vi "Write Pulse Recorder Configuration.vi"(8 "error in (no error)":errorcluster, 10 "Configuration":T1={"Pre-trigger duration"=0.01, "Post-trigger duration"=0.1, "Rate"=1000000.0, "Ranges"=[10.0], "Re-name channels"=[], "Active channels"="0:1", "External clock"=FALSE} {"Rate" format="%#_8pHz"; "Post-trigger duration" format="%#_6ps"; "Pre-trigger duration" format="%#_6ps"; "Ranges" format="%#_6pV"}, 11 "RP I-V in":refnum<class "RP I-V.lvclass">) -> (0 "error out":errorcluster, 3 "RP I-V out":refnum<class "RP I-V.lvclass">)   [LabVIEW 2016, in "RP I-V.lvclass"]
uses:
  RP I-V.lvclass
  NHMFL_Core/Libraries/Instruments/Pulse Driver/Pusle Driver Configuration.ctl
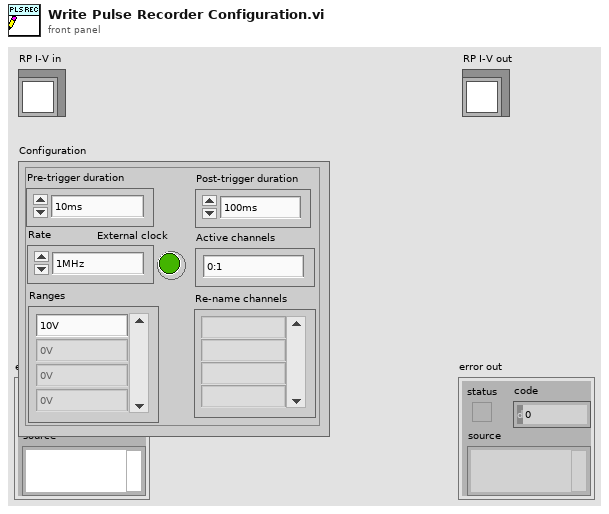
[diagram p1: front panel]
types:
  T1 = typedef "Pusle Driver Configuration.ctl" = cluster{"Pre-trigger duration":dbl, "Post-trigger duration":dbl, "Rate":dbl, "Ranges":dbl[], "Re-name channels":string[], "Active channels":string, "External clock":bool}
  T2 = typedef "RP I-V Configuration.ctl" = cluster{"Recorder":T1, "I-V parameters":T3}
  T3 = typedef "I-V parameters.ctl" = cluster{"Start magnitude":dbl, "Magnitude increment":dbl, "Number of pulses":i32, "Baseline length":dbl, "Ramp length":dbl, "Top  length":dbl, "Threshold ":dbl}
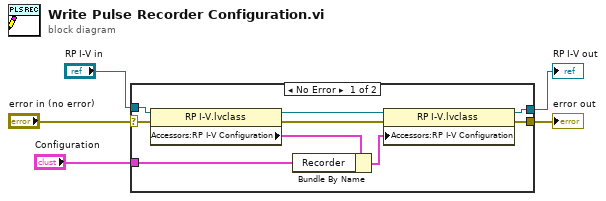
[diagram p0: block diagram]
diagram:
  n1 = case shown="No Error" "error in (no error)" {
    selector: "error in (no error)" -> [w6 w16]
    tunnel: [w8 w16] -> w2
    tunnel: "RP I-V in" -> [w12 w15]
    tunnel: "Configuration" -> [w10 _]
    tunnel: [w7 w15] -> w3
    frame No Error {
      n2 = property class="RP I-V.lvclass"(reference=w12, error in=w6) -> (reference out=w14:refnum<class "RP I-V.lvclass">, error out=w13:errorcluster, "Accessors:RP I-V Configuration"=w11:T2)
      n3 = Bundle By Name(cluster=w11, "Recorder"=w10) -> (w9:T2)
      n4 = property class="RP I-V.lvclass"(reference=w14, error in=w13, "Accessors:RP I-V Configuration"=w9) -> (reference out=w7:refnum<class "RP I-V.lvclass">, error out=w8:errorcluster)
    }
    frame Error {
    }
  }
  "error out" <- w2
  "RP I-V out" <- w3
